vi "Convert DIDPID Parameters Array to String Array.vi"(8 "error in (no error)":errorcluster, 11 "PID Parameters":T1[](array[typedef]) {"Byte Order" items=["Little Endian", "Big Endian"]; "Data Type" items=["Signed", "Unsigned", "IEEE Float"]}) -> (0 "error out":errorcluster, 3 "PID Parameters":string[][](array[string]))   [LabVIEW 2015, in "Diagnostics Addon System Explorer.lvlib"]
uses:
  Diagnostics Addon System Explorer.lvlib
  Shared/DIDPID Signal Parameters.ctl
  Shared/Diagnostics Addon Shared.lvlib
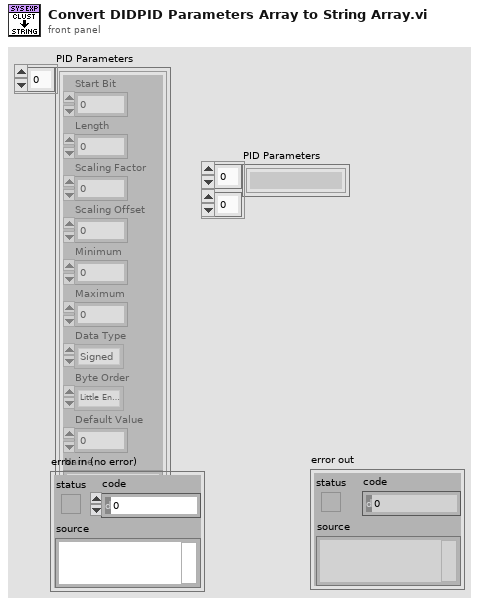
[diagram p1: front panel]
types:
  T1 = typedef "Diagnostics Addon Shared.lvlib/DIDPID Signal Parameters.ctl" = cluster{"Start Bit":u8, "Length":u8, "Scaling Factor":dbl, "Scaling Offset":dbl, "Minimum":dbl, "Maximum":dbl, "Data Type":u32, "Byte Order":u32, "Default Value":dbl, "Name":string, "Units":string, "Description":string}
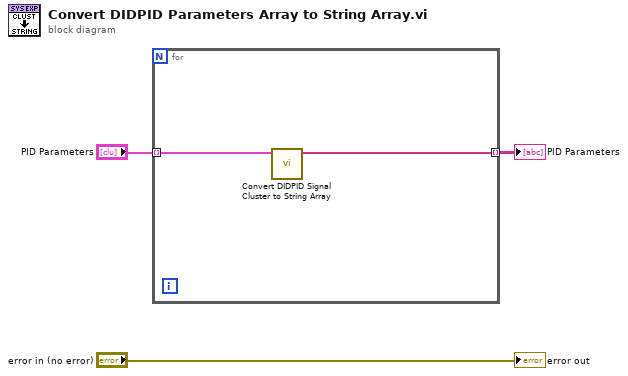
[diagram p0: block diagram]
diagram:
  n1 = for {
    tunnel: [w5] -> w3 mode=indexing
    tunnel: "PID Parameters" -> [w4] mode=indexing
    n2 = call "Convert DIDPID Signal Cluster to String Array.vi"("Signal Parameters"=w4) -> ("Array"=w5:string[])  [unwired: 10 in]
  }
  "PID Parameters" <- w3
  "error out" <- "error in (no error)"
